vi "Array to File.vi"(8 "error in":errorcluster, 10 "array in":T1[](array[typedef]) {"Creation Date" format="%<%x>T"; "Last Updated" format="%<%x>T"}, 11 "file path in":path) -> (0 "error out":errorcluster, 3 "file path out":path)   [LabVIEW 2018]
uses:
  Type Defs/SR Cluster.ctl
  Type Defs/SR Status.ctl
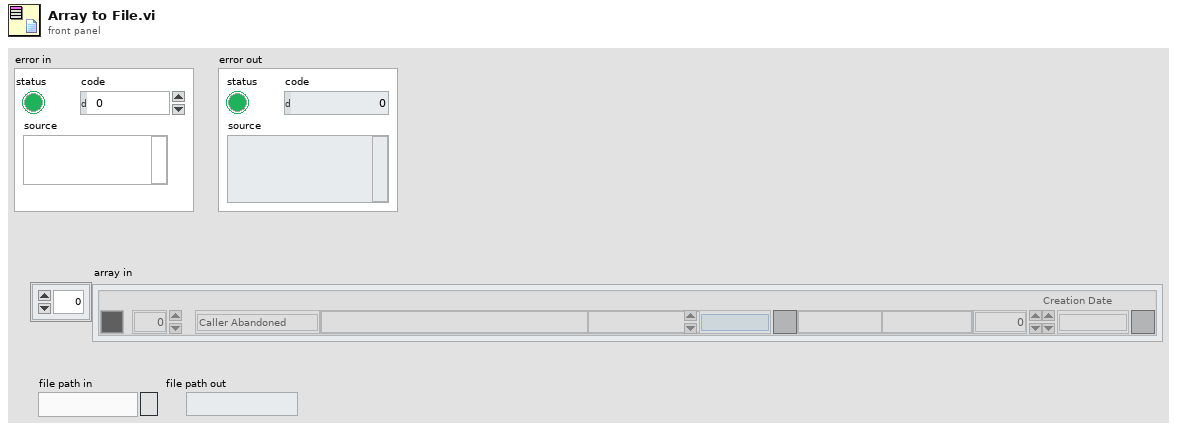
[diagram p1: front panel]
types:
  T1 = typedef "SR Cluster.ctl" = cluster{"Color":u32, "SR Number":i32, "SR Status":T2, "Name":string, "Summary":string, "Last Updated":timestamp, "SR Type":string, "Service Level":string, "Days Open":dbl, "Creation Date":timestamp}
  T2 = typedef "SR Status.ctl" = enum16{"Caller Abandoned", "Created in Error", "Expired", "Forum Resolved AE", "Forum Resolved Customer", "IN WORK", "IN WORK Collab with AES", "IN WORK Collab with PSE", "IN WORK Collab with SE", "IN WORK Customer Added Note", "IN WORK Escalation", "IN WORK Wait on Customer", "Open", "Potentially Resolved", "Presumed Resolved", "RMA Approved for Return", "Resolved", "Passed Off"}
  T3 = enum16{"open", "replace", "create", "open or create", "replace or create", "replace or create with confirmation"}
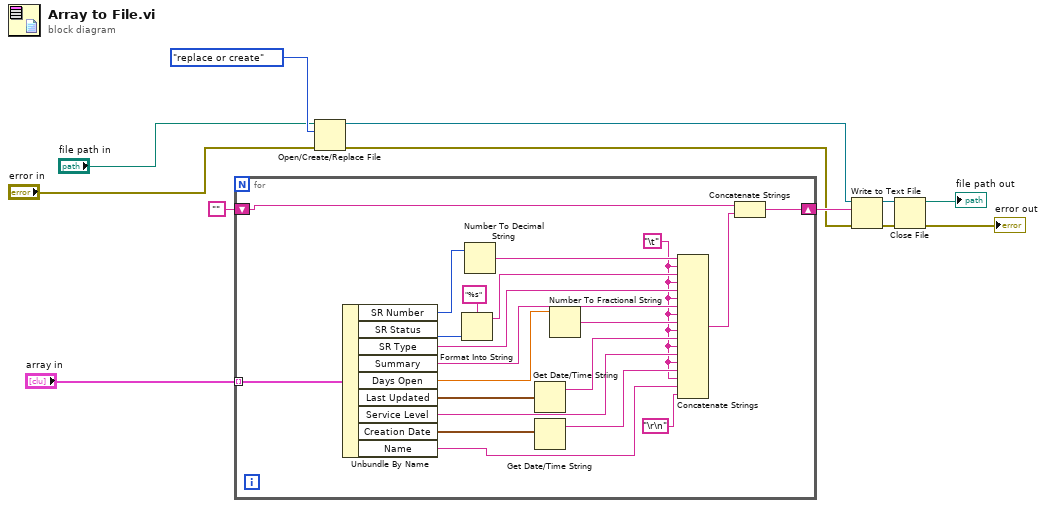
[diagram p0: block diagram]
diagram:
  n1 = for {
    shift-right: [w33] -> w10
    shift-left: "" -> [w32]
    tunnel: "array in" -> [w18] mode=indexing
    w15 = "\t"
    n2 = Unbundle By Name(w18) -> ("SR Number"=w30:i32, "SR Status"=w21:T2, "SR Type"=w28:string, "Summary"=w22:string, "Days Open"=w27:dbl, "Last Updated"=w23:timestamp, "Service Level"=w24:string, "Creation Date"=w17:timestamp, "Name"=w14:string)
    n3 = Format Into String(format string="%s", w21) -> (resulting string=w19:string)  [unwired: 2 in, 1 out]
    n4 = Number To Decimal String(number=w30) -> (decimal integer string=w29:string)  [unwired: 1 in]
    n5 = Get Date/Time String(seconds (now)=w23) -> (date string=w25:string)  [unwired: 2 in, 1 out]
    n6 = Get Date/Time String(seconds (now)=w17) -> (date string=w16:string)  [unwired: 2 in, 1 out]
    n7 = Number To Fractional String(number=w27) -> (F-format string=w26:string)  [unwired: 3 in]
    n8 = Concatenate Strings(w29, w15, w19, w15, w28, w15, w22, w15, w26, w15, w25, w15, w24, w15, w16, w15, w14, "\r\n") -> (w31:string)
    n9 = Concatenate Strings(w32, w31) -> (w33:string)
  }
  n10 = Open/Create/Replace File(file path (use dialog)="file path in", error in="error in", operation (0:open)=T3."replace or create") -> (refnum out=w8:refnum<file>, error out=w9:errorcluster)  [unwired: 3 in, 1 out]
  n11 = Write to Text File(file (use dialog)=w8, text=w10, error in=w9) -> (refnum out=w6:refnum<file>, error out=w7:errorcluster)  [unwired: 1 in, 1 out]
  n12 = Close File(refnum=w6, error in=w7) -> (path=→"file path out":path, error out=→"error out":errorcluster)
